vi "data to bytestream.vi"(9 "specifications":T1[](array[typedef]), 10 "byte allocation":u8[](array[numeric]), 11 "data table":T3) -> (2 "bytestream":u8[](array[numeric]), 3 "allocation":T3)   [LabVIEW 2013, in "EthernetIP runtime.lvclass"]
uses:
  EthernetIP runtime.lvclass
  <vilib>/NI/Tag Bus/table/data table.ctl
  conversion specification.ctl
  <vilib>/NI/Tag Bus/tag/Data Type.ctl
  <vilib>/NI/Tag Bus/table/data polymorphs/read one/read Double.vi
  <vilib>/NI/Tag Bus/table/data polymorphs/read one/read Single.vi
  <vilib>/NI/Tag Bus/table/data polymorphs/read one/read I64.vi
  <vilib>/NI/Tag Bus/table/data polymorphs/read one/read U64.vi
  <vilib>/NI/Tag Bus/table/data polymorphs/read one/read I32.vi
  <vilib>/NI/Tag Bus/table/data polymorphs/read one/read U32.vi
  <vilib>/NI/Tag Bus/table/data polymorphs/read one/read I16.vi
  <vilib>/NI/Tag Bus/table/data polymorphs/read one/read U16.vi
  <vilib>/NI/Tag Bus/table/data polymorphs/read one/read I8.vi
  <vilib>/NI/Tag Bus/table/data polymorphs/read one/read U8.vi
  <vilib>/NI/Tag Bus/table/data polymorphs/read one/read Boolean.vi
  <vilib>/NI/Tag Bus/table/data table.lvlib
  <vilib>/NI/Tag Bus/tag/tag descriptor.lvclass
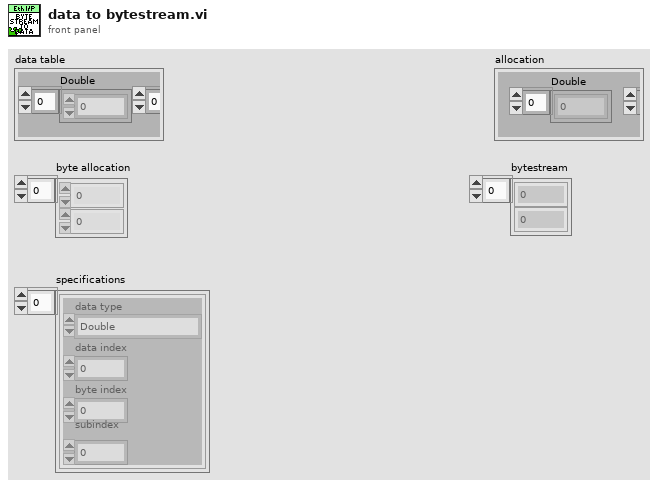
[diagram p1: front panel]
types:
  T1 = typedef "EthernetIP runtime.lvclass/conversion specification.ctl" = cluster{"data type":T2, "data index":i32, "byte index":i32, "subindex":i32}
  T2 = typedef "tag bus.lvlib/tag descriptor.lvclass/Data Type.ctl" = enum16{"Double", "Single", "I64", "I32", "I16", "I8", "U64", "U32", "U16", "U8", "Boolean", "String", "Array of Double", "Array of Single", "Array of I64", "Array of I32", "Array of I16", "Array of I8", "Array of U64", "Array of U32", "Array of U16", "Array of U8", "Array of Boolean", "Array of String"}
  T3 = typedef "tag bus.lvlib/data table.lvlib/data table.ctl" = cluster{"Double":dbl[], "Single":sgl[], "I64":i64[], "I32":i32[], "I16":i16[], "I8":i8[], "U64":u64[], "U32":u32[], "U16":u16[], "U8":u8[], "Boolean":bool[], "String":string[], "Array of Double":cluster{"DBL Array":dbl[]}[], "Array of Single":cluster{"SGL Array":sgl[]}[], "Array of I64":cluster{"I64 Array":i64[]}[], "Array of I32":cluster{"I32 Array":i32[]}[], "Array of I16":cluster{"I16 Array":i16[]}[], "Array of I8":cluster{"I8 Array":i8[]}[], "Array of U64":cluster{"U64 Array":u64[]}[], "Array of U32":cluster{"U32 Array":u32[]}[], "Array of U16":cluster{"U16 Array":u16[]}[], "Array of U8":cluster{"U8 Array":u8[]}[], "Array of Boolean":cluster{"Boolean Array":bool[]}[], "Array of String":cluster{"String Array":string[]}[]}
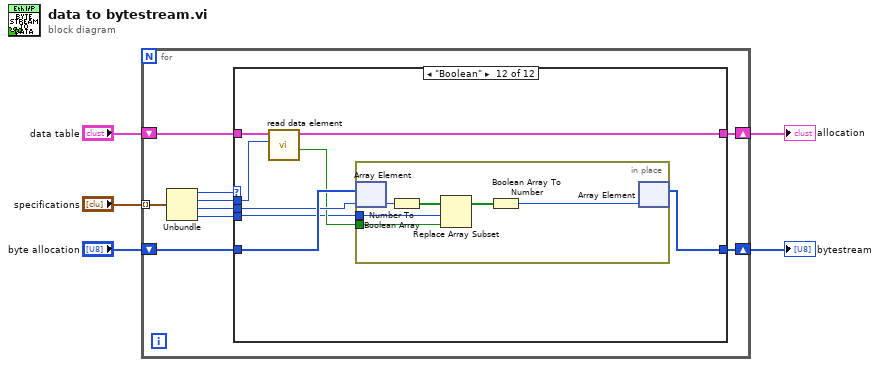
[diagram p0: block diagram]
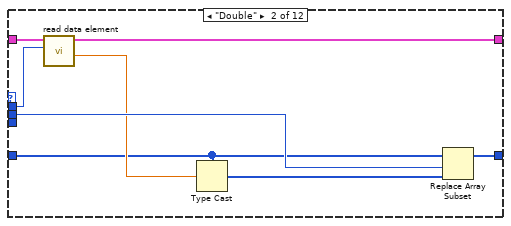
[diagram p3: hidden frame]
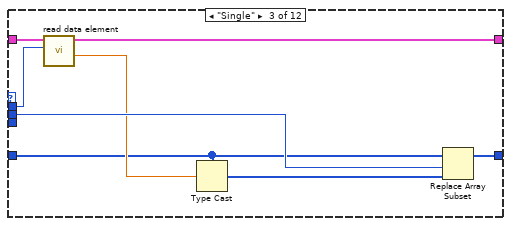
[diagram p4: hidden frame]
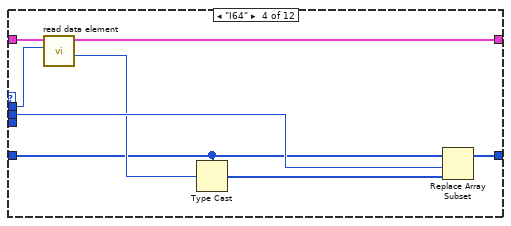
[diagram p5: hidden frame]
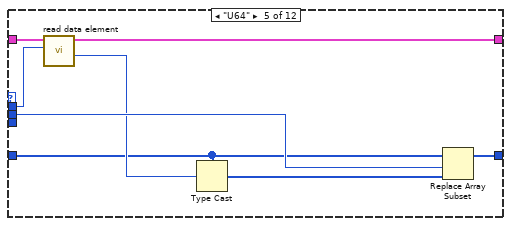
[diagram p6: hidden frame]
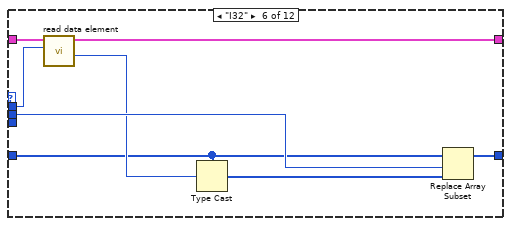
[diagram p7: hidden frame]
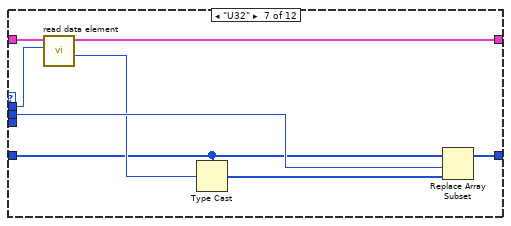
[diagram p8: hidden frame]
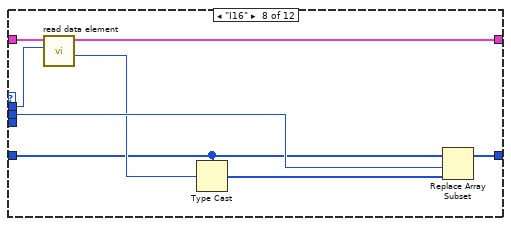
[diagram p9: hidden frame]
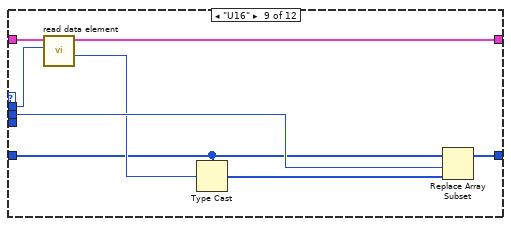
[diagram p10: hidden frame]
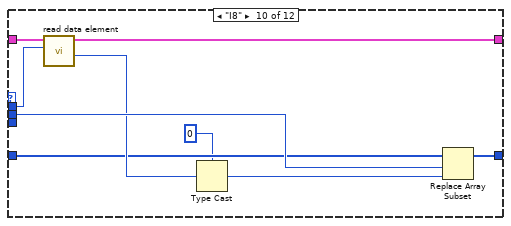
[diagram p11: hidden frame]
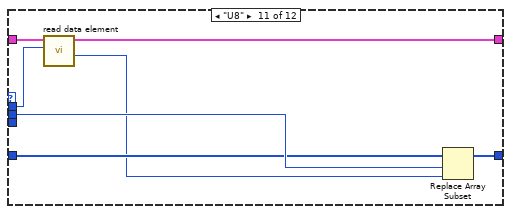
[diagram p12: hidden frame]
diagram:
  n1 = for {
    shift-right: [w11] -> w4
    shift-left: "data table" -> [w12]
    tunnel: "specifications" -> [w14] mode=indexing
    shift-right: [w7] -> w1
    shift-left: "byte allocation" -> [w10]
    n2 = Unbundle(w14) -> ("data type"=w13:T2, "data index"=w9:i32, "byte index"=w6:i32, "subindex"=w8:i32)
    n3 = case shown="\"Boolean\"" w13 {
      tunnel: w12 -> [w16 w24 w32 w40 w48 w56 w64 w72 w80 w89 w96 w104]
      tunnel: [w16 w23 w31 w39 w47 w55 w63 w71 w79 w88 w95 w103] -> w11
      tunnel: w6 -> [_ w20 w28 w36 w44 w52 w60 w68 w76 w85 w92 w99]
      tunnel: w10 -> [w15 w18 w26 w34 w42 w50 w58 w66 w74 w83 w91 w101]
      tunnel: w9 -> [_ w22 w30 w38 w46 w54 w62 w70 w78 w87 w94 w102]
      tunnel: w8 -> [_ _ _ _ _ _ _ _ _ _ _ w97]
      tunnel: [w15 w21 w29 w37 w45 w53 w61 w69 w77 w86 w93 w100] -> w7
      frame Default {
      }
      frame "Double" {
        n4 = call-poly <vilib>:"read data element.vi"("index"=w22, "data table in"=w24) -> ("value"=w19:dbl, "data table out"=w23:T3)  [unwired: 8 in]
        n5 = Type Cast(type=w18, x=w19) -> (*(type *) &x=w17:u8[])
        n6 = Replace Array Subset(array=w18, new element=w17, index=w20) -> (w21:u8[])
      }
      frame "Single" {
        n7 = call-poly <vilib>:"read data element.vi"("index"=w30, "data table in"=w32) -> ("value"=w27:sgl, "data table out"=w31:T3)  [unwired: 8 in]
        n8 = Type Cast(type=w26, x=w27) -> (*(type *) &x=w25:u8[])
        n9 = Replace Array Subset(array=w26, new element=w25, index=w28) -> (w29:u8[])
      }
      frame "I64" {
        n10 = call-poly <vilib>:"read data element.vi"("index"=w38, "data table in"=w40) -> ("value"=w35:i64, "data table out"=w39:T3)  [unwired: 8 in]
        n11 = Type Cast(type=w34, x=w35) -> (*(type *) &x=w33:u8[])
        n12 = Replace Array Subset(array=w34, new element=w33, index=w36) -> (w37:u8[])
      }
      frame "U64" {
        n13 = call-poly <vilib>:"read data element.vi"("index"=w46, "data table in"=w48) -> ("value"=w43:u64, "data table out"=w47:T3)  [unwired: 8 in]
        n14 = Type Cast(type=w42, x=w43) -> (*(type *) &x=w41:u8[])
        n15 = Replace Array Subset(array=w42, new element=w41, index=w44) -> (w45:u8[])
      }
      frame "I32" {
        n16 = call-poly <vilib>:"read data element.vi"("index"=w54, "data table in"=w56) -> ("value"=w51:i32, "data table out"=w55:T3)  [unwired: 8 in]
        n17 = Type Cast(type=w50, x=w51) -> (*(type *) &x=w49:u8[])
        n18 = Replace Array Subset(array=w50, new element=w49, index=w52) -> (w53:u8[])
      }
      frame "U32" {
        n19 = call-poly <vilib>:"read data element.vi"("index"=w62, "data table in"=w64) -> ("value"=w59:u32, "data table out"=w63:T3)  [unwired: 8 in]
        n20 = Type Cast(type=w58, x=w59) -> (*(type *) &x=w57:u8[])
        n21 = Replace Array Subset(array=w58, new element=w57, index=w60) -> (w61:u8[])
      }
      frame "I16" {
        n22 = call-poly <vilib>:"read data element.vi"("index"=w70, "data table in"=w72) -> ("value"=w67:i16, "data table out"=w71:T3)  [unwired: 8 in]
        n23 = Type Cast(type=w66, x=w67) -> (*(type *) &x=w65:u8[])
        n24 = Replace Array Subset(array=w66, new element=w65, index=w68) -> (w69:u8[])
      }
      frame "U16" {
        n25 = call-poly <vilib>:"read data element.vi"("index"=w78, "data table in"=w80) -> ("value"=w75:u16, "data table out"=w79:T3)  [unwired: 8 in]
        n26 = Type Cast(type=w74, x=w75) -> (*(type *) &x=w73:u8[])
        n27 = Replace Array Subset(array=w74, new element=w73, index=w76) -> (w77:u8[])
      }
      frame "I8" {
        n28 = call-poly <vilib>:"read data element.vi"("index"=w87, "data table in"=w89) -> ("value"=w84:i8, "data table out"=w88:T3)  [unwired: 8 in]
        n29 = Type Cast(type=u8 0, x=w84) -> (*(type *) &x=w82:u8)
        n30 = Replace Array Subset(array=w83, new element=w82, index=w85) -> (w86:u8[])
      }
      frame "U8" {
        n31 = call-poly <vilib>:"read data element.vi"("index"=w94, "data table in"=w96) -> ("value"=w90:u8, "data table out"=w95:T3)  [unwired: 8 in]
        n32 = Replace Array Subset(array=w91, new element=w90, index=w92) -> (w93:u8[])
      }
      frame "Boolean" {
        n33 = call-poly <vilib>:"read data element.vi"("index"=w102, "data table in"=w104) -> ("value"=w98:bool, "data table out"=w103:T3)  [unwired: 8 in]
        n34 = in-place {
          in-place-border: w98 -> [w106]
          in-place-border: w97 -> [w105]
          n35 = in-place-array #1(w101, w99) -> (w110:u8)
          n36 = Number To Boolean Array(number=w110) -> (Boolean array=w108:bool[])
          n37 = Replace Array Subset(array=w108, new element=w106, index=w105) -> (w107:bool[])
          n38 = Boolean Array To Number(Boolean array=w107) -> (number=w109:u8)
          n39 = in-place-array #1(w109) -> (w100:u8[])  [unwired: 1 out]
        }
      }
    }
  }
  "allocation" <- w4
  "bytestream" <- w1
